vi "Test MQTT-3.14.4-1.vi"(8 "error in (no error)":errorcluster) -> (0 "error out":errorcluster)   [LabVIEW 2013]
uses:
  source/Client/Client.lvclass
  <vilib>/addons/_JKI Toolkits/Caraya/classes/Test/Test.lvclass
  <vilib>/addons/_JKI Toolkits/Caraya/classes/Assert/Assert.lvclass
  source/MQTT_Base/MQTT_Base.lvclass
  source/Control Packets/DISCONNECT/DISCONNECT.lvclass
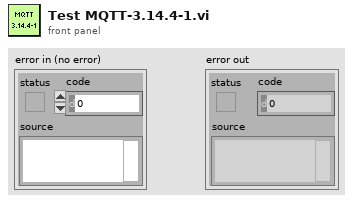
[diagram p1: front panel]
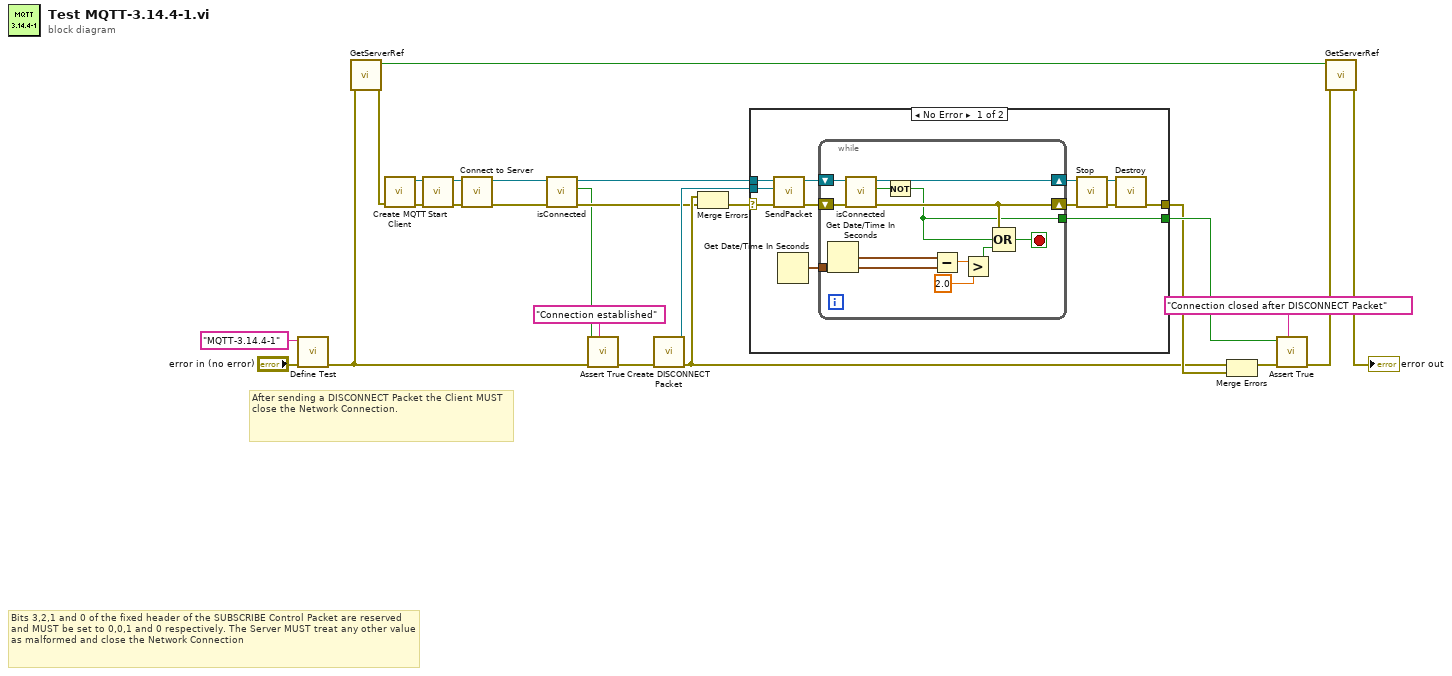
[diagram p0: block diagram]
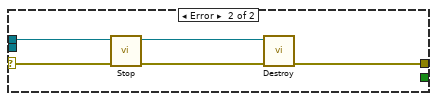
[diagram p2: hidden frame]
diagram:
  # "After sending a DISCONNECT Packet the Client MUST close the Network Connection."
  # "Bits 3,2,1 and 0 of the fixed header of the SUBSCRIBE Control Packet are reserved and MUST be set to 0,0,1 and 0 respectively. The Server MUST treat any other value as malformed and close the Network Connection"
  n1 = call <vilib>:"Define Test.vi"("error in (no error)"="error in (no error)", "Label (VI Title)"="MQTT-3.14.4-1") -> ("error out"=w3:errorcluster)  [unwired: 9 in]
  n2 = call "GetServerRef.vi"("error in"=w3) -> ("error out"=w22:errorcluster, "Created"=w23:bool)  [unwired: 8 in, 1 out]
  n3 = call "Create MQTT Client.vi"("error in (no error)"=w22) -> ("error out"=w12:errorcluster, "Client out"=w14:refnum<class "Client.lvclass">)  [unwired: 9 in]
  n4 = call "Start.vi"("error in (no error)"=w12, "MQTT_Base in"=w14) -> ("error out"=w11:errorcluster, "MQTT_Base out"=w13:refnum<class "Client.lvclass">)  [unwired: 7 in, 1 out]
  n5 = call "Connect to Server.vi"("error in (no error)"=w11, "Client in"=w13) -> ("error out"=w8:errorcluster, "Client out"=w6:refnum<class "Client.lvclass">)  [unwired: 7 in, 1 out]
  n6 = call "isConnected.vi"("error in (no error)"=w8, "Client in"=w6) -> ("error out"=w7:errorcluster, "connected"=w1:bool, "Client out"=w5:refnum<class "Client.lvclass">)  [unwired: 7 in]
  n7 = call <vilib>:"Assert True.vi"("Label"="Connection established", "error in (no error)"=w3, "True?"=w1) -> ("error out"=w2:errorcluster)  [unwired: 8 in]
  n8 = call "Create DISCONNECT Packet.vi"("error in (no error)"=w2) -> ("error out"=w9:errorcluster, "DISCONNECT"=w10:refnum<class "DISCONNECT.lvclass">)  [unwired: 9 in]
  n9 = Merge Errors(w9, w7) -> (w15:errorcluster)
  n10 = case shown="No Error" w15 {
    selector: w15 -> [w35 w51]
    tunnel: w5 -> [w36 w53]
    tunnel: [w37 w54] -> w16
    tunnel: [w31 _] -> w18
    tunnel: w10 -> [w34 _]
    frame No Error {
      n11 = call "SendPacket.vi"("error in (no error)"=w35, "ControlPacket"=w34, "Client in"=w36) -> ("error out"=w32:errorcluster, "Client out"=w33:refnum<class "Client.lvclass">)  [unwired: 6 in, 1 out]
      n12 = Get Date/Time In Seconds() -> (seconds since 1Jan1904=w30:timestamp)
      n13 = while {
        shift-right: [w46] -> w27
        shift-left: w32 -> [w47]
        shift-right: [w48] -> w29
        shift-left: w33 -> [w49]
        tunnel: [w43] -> w31
        tunnel: w30 -> [w38]
        stop <- w45 stop-if-true
        n14 = Get Date/Time In Seconds() -> (seconds since 1Jan1904=w42:timestamp)
        n15 = call "isConnected.vi"("error in (no error)"=w47, "Client in"=w49) -> ("error out"=w46:errorcluster, "connected"=w44:bool, "Client out"=w48:refnum<class "Client.lvclass">)  [unwired: 7 in]
        n16 = Not(x=w44) -> (.not. x?=w43:bool)
        n17 = Subtract(x=w42, y=w38) -> (x-y=w41:dbl)
        n18 = Greater?(x=w41, y=2.0) -> (0:w39:bool)
        n19 = Compound Arithmetic op=OR(w46, w43, w39) -> (w45:bool)
      }
      n20 = call "Stop.vi"("error in (no error)"=w27, "MQTT_Base in"=w29) -> ("error out"=w26:errorcluster, "MQTT_Base out"=w28:refnum<class "Client.lvclass">)  [unwired: 7 in, 1 out]
      n21 = call-dynamic "Destroy.vi"("error in (no error)"=w26, "Client in"=w28) -> ("error out"=w37:errorcluster)  [unwired: 8 in, 1 out]
    }
    frame Error {
      n22 = call "Stop.vi"("error in (no error)"=w51, "MQTT_Base in"=w53) -> ("error out"=w50:errorcluster, "MQTT_Base out"=w52:refnum<class "Client.lvclass">)  [unwired: 7 in, 1 out]
      n23 = call-dynamic "Destroy.vi"("error in (no error)"=w50, "Client in"=w52) -> ("error out"=w54:errorcluster)  [unwired: 8 in, 1 out]
    }
  }
  n24 = Merge Errors(w9, w16) -> (w17:errorcluster)
  n25 = call <vilib>:"Assert True.vi"("Label"="Connection closed after DISCONNECT Packet", "error in (no error)"=w17, "True?"=w18) -> ("error out"=w21:errorcluster)  [unwired: 8 in]
  n26 = call "GetServerRef.vi"("error in"=w21, "Destroy (F)"=w23) -> ("error out"=→"error out":errorcluster)  [unwired: 7 in, 2 out]
